vi "Init User Prefs.vi"(8 "error in (no error)":errorcluster, 11 "Historian Charting Manager in":refnum<class "Historian Charting Manager.lvclass">) -> (0 "error out":errorcluster, 3 "Historian Charting Manager out":refnum<class "Historian Charting Manager.lvclass">)   [LabVIEW 2020, in "VolatusGUI.lvlib" / "Historian Charting Manager.lvclass"]
uses:
  Historian Charting Manager.lvclass
  Historian Charting Manager.lvclass/Historian Charting Manager.ctl
  lv-userprefs/User Prefs/PrefsDB/PrefsDB.lvclass
  lv-userprefs/User Prefs/Pref Group/Pref Group.lvclass
  Volatus/Module/Module.lvclass
  C:/dev/lv20CE/relink/lv-volatus/Volatus/Module/Module.lvclass
  C:/dev/lv20CE/relink/lv-volatus/VolatusGUI/Historian Charting Manager/Historian Charting Manager.lvclass
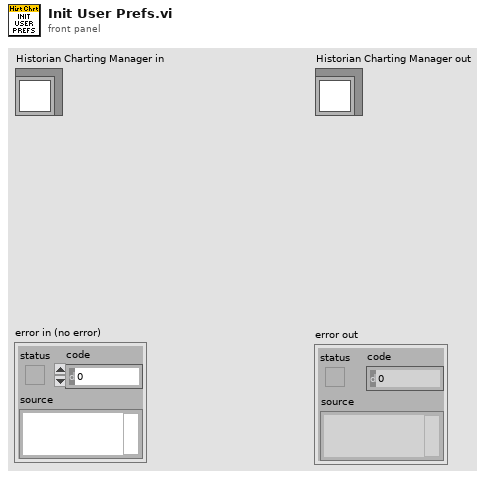
[diagram p1: front panel]
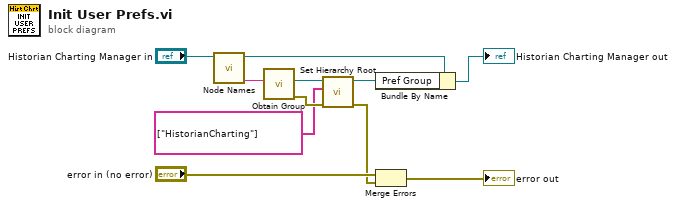
[diagram p0: block diagram]
diagram:
  n1 = call "Node Names.vi"("Module in"="Historian Charting Manager in") -> ("Node"=w5:string, "Module out"=w6:refnum<class "Historian Charting Manager.lvclass">)  [unwired: 6 in, 3 out]
  n2 = call "Obtain Group.vi"("Group"=w5) -> ("error out"=w9:errorcluster, "Pref Group"=w10:refnum<class "Pref Group.lvclass">)  [unwired: 8 in, 1 out]
  n3 = call "Set Hierarchy Root.vi"("error in (no error)"=w9, "Hierarchy Root"=string[] ["HistorianCharting"], "Pref Group in"=w10) -> ("error out"=w3:errorcluster, "Pref Group out"=w1:refnum<class "Pref Group.lvclass">)  [unwired: 7 in]
  n4 = Bundle By Name(cluster=w6, "Pref Group"=w1) -> (→"Historian Charting Manager out":refnum<class "Historian Charting Manager.lvclass">)
  n5 = Merge Errors("error in (no error)", w3) -> (→"error out":errorcluster)
